vi "AddADCWSEQ.vi"(0 "VISA resource name":refnum<visa-resource-name>, 1 "Test Mode":string(combo)="ACW", 2 "Test Voltage (V)":string, 3 "Ramp Time (s)":string, 4 "Dwell Time (s)":string, 5 "Min Leakag (A)":string, 6 "Max Leakage (A)":string, 7 "error in (no error)":errorcluster, 8 "Sequence Number":string, 9 "DUT Type I":string(combo)="Isolated DUT", 10 "Sequence Name":string, 11 "DUT Type II (DCW Only)":string(combo)="Resistive DUT") -> (20 "VISA resource name out":refnum<visa-resource-name>, 25 "Error Message":string, 26 "Error Code":i32, 27 "error out":errorcluster)   [LabVIEW 2010, in "VITREK V7X.lvlib"]
doc: "Add a AC/DCW test step into a sequence and save this sequence into the requested store number."
uses:
  VITREK V7X.lvlib
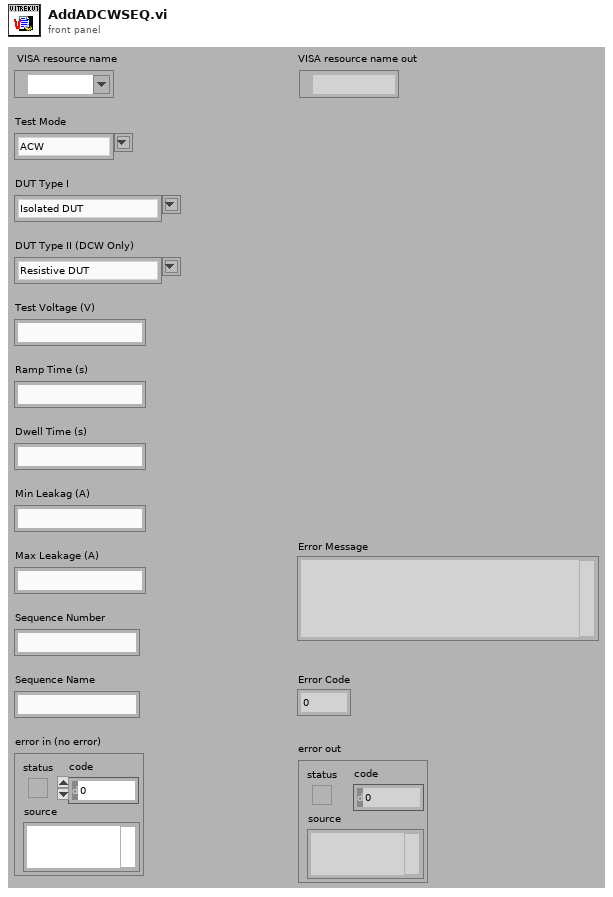
[diagram p1: front panel]
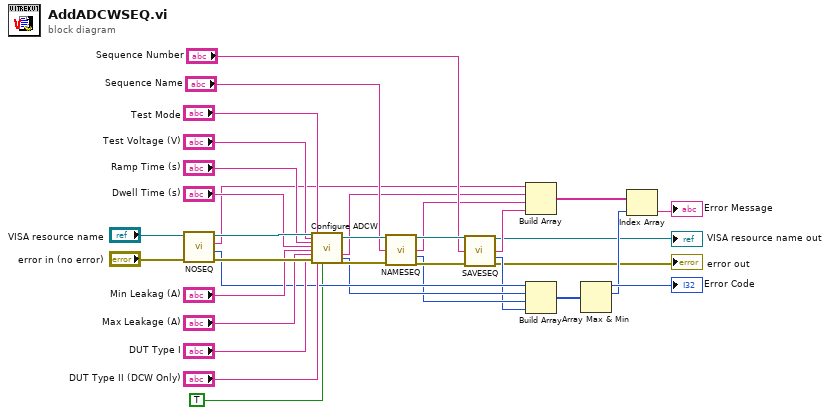
[diagram p0: block diagram]
diagram:
  n1 = call "NOSEQ.vi"("error in (no error)"="error in (no error)", "VISA resource name"="VISA resource name") -> ("error out"=w31:errorcluster, "Error Code"=w7:i32, "Error Message"=w11:string, "VISA resource name out"=w32:refnum<visa-resource-name>)  [unwired: 6 in]
  n2 = call "Configure ADCW.vi"("VISA resource name"=w32, "Test Voltage (V)"="Test Voltage (V)", "Ramp Time (s)"="Ramp Time (s)", "Dwell Time (s)"="Dwell Time (s)", "Min Leakag (A)"="Min Leakag (A)", "Max Leakage (A)"="Max Leakage (A)", "DUT Type I"="DUT Type I", "error in (no error)"=w31, "Test Mode"="Test Mode", "DUT Type II (DCW Only)"="DUT Type II (DCW Only)", "Command Terminator"=TRUE) -> ("VISA resource name out"=w29:refnum<visa-resource-name>, "Error Message"=w10:string, "Error Code"=w6:i32, "error out"=w30:errorcluster)  [unwired: 12 in, 1 out]
  n3 = call "NAMESEQ.vi"("VISA resource name"=w29, "Sequence Name"="Sequence Name", "error in (no error)"=w30) -> ("VISA resource name out"=w27:refnum<visa-resource-name>, "Error Message"=w9:string, "Error Code"=w5:i32, "error out"=w28:errorcluster)  [unwired: 9 in]
  n4 = call "SAVESEQ.vi"("VISA resource name"=w27, "Sequence Number"="Sequence Number", "error in (no error)"=w28) -> ("VISA resource name out"=→"VISA resource name out":refnum<visa-resource-name>, "Error Message"=w8:string, "Error Code"=w4:i32, "error out"=→"error out":errorcluster)  [unwired: 9 in]
  n5 = Build Array(w11, w10, w9, w8) -> (w16:string[])
  n6 = Build Array(w7, w6, w5, w4) -> (w14:i32[])
  n7 = Array Max & Min(array=w14) -> (max value=→"Error Code":i32, max index (indices)=w12:i32)  [unwired: 2 out]
  n8 = Index Array(array=w16, index=w12) -> (element=→"Error Message":string)
